vi "Differential_delay_line_Mezzaninev56.vi"() -> ()   [LabVIEW 2009]
panel:
  in  "channel":i32
  out "error out 2":errorcluster
  in  "Delay value":u16
  in  "Id in":i32
  in  "error in (no error)":errorcluster
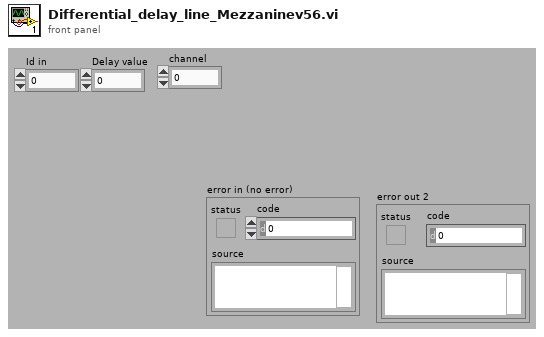
[diagram p1: front panel]
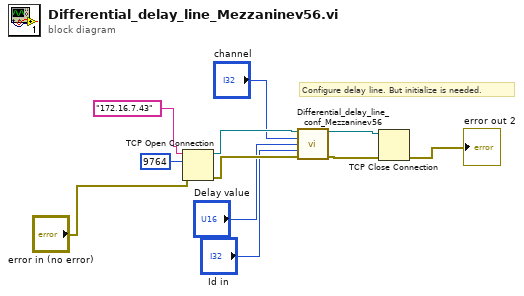
[diagram p0: block diagram]
diagram:
  # "Configure delay line. But initialize is needed."
  n1 = TCP Open Connection(address="172.16.7.43", remote port or service name=u16 9764, error in (no error)="error in (no error)") -> (connection ID=w7:refnum<k5>, error out=w9:errorcluster)  [unwired: 2 in]
  n2 = call "Differential_delay_line_conf_Mezzaninev56.vi"("connection ID"=w7, "channel"="channel", "Delay value"="Delay value", "Id in"="Id in", "error in (no error)"=w9) -> ("connection ID out"=w2:refnum<k5>, "error out 2"=w3:errorcluster)  [unwired: 3 in, 6 out]
  n3 = TCP Close Connection(connection ID=w2, error in (no error)=w3) -> (error out=→"error out 2":errorcluster)  [unwired: 1 in, 1 out]
